vi "Describe Call Comparison.vi"(10 "VI Call 2":refnum<class "VI Call.lvclass">, 11 "VI Call in":refnum<class "VI Call.lvclass">) -> (3 "delimited string":string)   [LabVIEW 2020, in "Identical Inputs Comparator.lvclass"]
uses:
  Identical Inputs Comparator.lvclass
  Core/VI Call/VI Call.lvclass
  Core/Comparator/Describe Variant.vi
  astemes-string-diff-utils/source/Diff Tool.vi
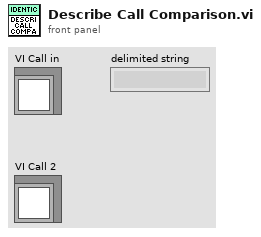
[diagram p1: front panel]
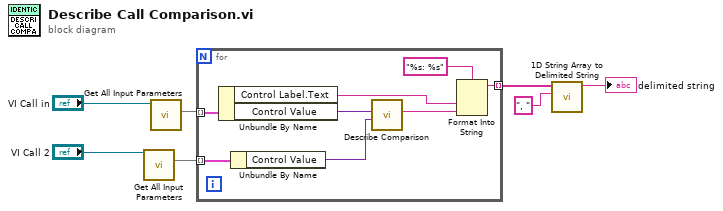
[diagram p0: block diagram]
diagram:
  n1 = call-dynamic "Get All Input Parameters.vi"("VI Call in"="VI Call 2") -> ("Input Parameters"=w6:map{string, variant})  [unwired: 9 in, 1 out]
  n2 = call-dynamic "Get All Input Parameters.vi"("VI Call in"="VI Call in") -> ("Input Parameters"=w4:map{string, variant})  [unwired: 9 in, 1 out]
  n3 = for {
    tunnel: w4 -> [w15] mode=indexing
    tunnel: w6 -> [w14] mode=indexing
    tunnel: [w8] -> w1 mode=indexing
    n4 = Unbundle By Name(w15) -> ("Control Label.Text"=w9:string, "Control Value"=w13:variant)
    n5 = Unbundle By Name(w14) -> ("Control Value"=w12:variant)
    n6 = call "Describe Comparison.vi"("Control Value 2"=w12, "Control Value 1"=w13) -> ("Description"=w10:string)  [unwired: 8 in, 1 out]
    n7 = Format Into String(format string="%s: %s", w9, w10) -> (resulting string=w8:string)  [unwired: 2 in, 1 out]
  }
  n8 = call <vilib>:"1D String Array to Delimited String.vi"("delimiter"=", ", "string array"=w1) -> ("delimited string"=→"delimited string":string)  [unwired: 9 in]
